vi "StopMotors.vi"(0 "handle in":i32, 1 "UnitAddress(0)":u16, 5 "error in":errorcluster, 7 "Motors":T1) -> (14 "handle out":i32, 19 "error out":errorcluster)   [LabVIEW 2014, in "Sixpack - Driver.lvlib"]
doc: "Mehrere Motoren können gemeinsam abgebremst werden, indem über dieses Kommando die Zielposition mit der aktuellen Position gleichgesetzt wird. Die Motoren werden dennoch mit der in AMax festgelegten negativen Beschleunigung abgebremst.\n\nCMD $2A\nMask: Maske für Abbremsen\n(OFF: Motor ausmaskiert, ON: Zielposition auf aktuelle Position setzen)"
uses:
  Sixpack - Driver.lvlib
  DLL/PackDLL.dll
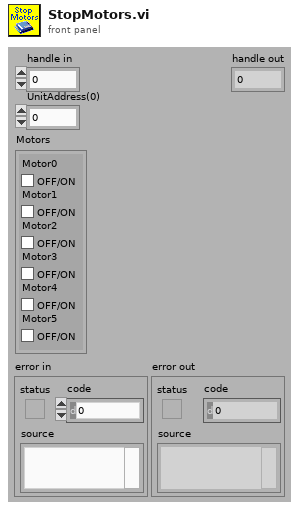
[diagram p1: front panel]
types:
  T1 = cluster{"Motor0":bool, "Motor1":bool, "Motor2":bool, "Motor3":bool, "Motor4":bool, "Motor5":bool}
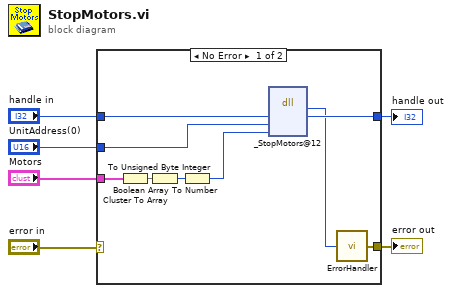
[diagram p0: block diagram]
diagram:
  n1 = case shown="No Error" "error in" {
    selector: "error in" -> [_ w16]
    tunnel: "handle in" -> [w15 w17]
    tunnel: [w14 w17] -> w5
    tunnel: "UnitAddress(0)" -> [w13 _]
    tunnel: "Motors" -> [w10 _]
    tunnel: [w8 w16] -> w2
    frame No Error {
      n2 = Cluster To Array(cluster=w10) -> (array=w11:bool[])
      n3 = Boolean Array To Number(Boolean array=w11) -> (number=w12:u32)
      n4 = To Unsigned Byte Integer(number=w12) -> (unsigned 8bit integer=w9:u8)
      n5 = dll-call lib="D:/CS-Source/LV2014/GPL/instr.lib/SixPack/PackDLL/DLL/PackDLL.dll" fn="_StopMotors@12" label="StopMotors"("HANDLE"=w15, "UnitAddress"=w13, "Mask"=w9) -> ("BOOLEAN"=w7:i8, "HANDLE"=w14:i32)  [unwired: 5 in, 2 out]
      n6 = call "ErrorHandler.vi"("BOOLEAN"=w7) -> ("error out"=w8:errorcluster)
    }
    frame Error {
    }
  }
  "handle out" <- w5
  "error out" <- w2
